vi "createTimestamp.vi"(8 "error in (no error)":errorcluster, 11 "Boot in":refnum<class "Boot.lvclass">) -> (0 "error out":errorcluster, 2 "Timestamp":refnum<class "Timestamp.lvclass">, 3 "Boot out":refnum<class "Boot.lvclass">)   [LabVIEW 2016, in "Boot.lvclass"]
uses:
  Boot.lvclass
  Common_RT_Timestamp/Timestamp/Timestamp.lvclass
  Resources/TimestampControlFIFO/TimestampControlFIFO.lvclass
  D:/Code/ts_M1M3Support/Common_RT_FPGA/IWriteU64FIFO/IWriteU64FIFO.lvclass
  Boot.lvclass/Boot.ctl
  Resources/TimestampControlFIFO/TimestampControlFIFO.lvclass/TimestampControlFIFO.ctl
  Common_RT_Timestamp/Timestamp/Timestamp.lvclass/Timestamp.ctl
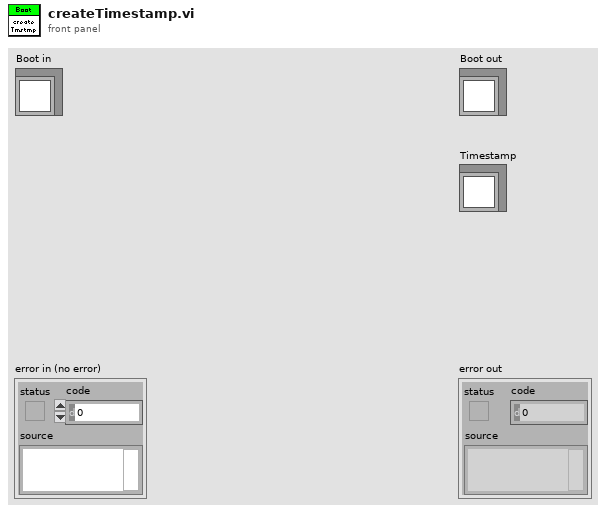
[diagram p1: front panel]
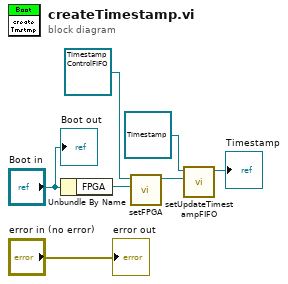
[diagram p0: block diagram]
diagram:
  n1 = Unbundle By Name("Boot in") -> ("FPGA"=w1:refnum<class "FPGA.lvclass">)
  n2 = call "setFPGA.vi"("FPGA"=w1, "TimestampControlFIFO in"=refnum<class "TimestampControlFIFO.lvclass"> refnum ("TimestampControlFIFO.lvclass")) -> ("TimestampControlFIFO out"=w2:refnum<class "TimestampControlFIFO.lvclass">)  [unwired: 9 in]
  n3 = call "setUpdateTimestampFIFO.vi"("UpdateTimestampFIFO"=w2, "Timestamp in"=refnum<class "Timestamp.lvclass"> refnum ("RTTimestamp.lvlib:Timestamp.lvclass")) -> ("Timestamp out"=→"Timestamp":refnum<class "Timestamp.lvclass">)  [unwired: 9 in]
  "error out" <- "error in (no error)"
  "Boot out" <- "Boot in"
